vi "Verify and Check-In.vi"(0 "File Data Manager in":refnum<class "File Data Manager.lvclass">, 5 "Rooms Manager GUID":string, 7 "Room No":string, 9 "Guest Contact Number In":string caption="Guest Contact Number", 11 "error in (no error)":errorcluster, 12 "Primary Guest Name":string, 13 "Adults":u32, 14 "Children":u32) -> (4 "File Data Manager out":refnum<class "File Data Manager.lvclass">, 15 "error out":errorcluster)   [LabVIEW 2023, in "File Data Manager.lvlib" / "File Data Manager.lvclass"]
uses:
  File Data Manager.lvclass
  C:/Program Files/National Instruments/LabVIEW 2023/vi.lib/ActorFramework/Actor/Actor.lvclass
  File Data Manager.lvclass/File Data Manager.ctl
  Central Data Manager/Central Data Manager/Room Occupancy Status.ctl
  <vilib>/ActorFramework/Actor/Actor.lvclass/Actor.ctl
  <vilib>/ActorFramework/Message Enqueuer/Message Enqueuer.lvclass/Message Enqueuer.ctl
  Interfaces/Incoming Hotel Management Tool Model Interface Messages/Update Check-in Status Msg/Update Check-in Status Msg.lvclass/Update Check-in Status Msg.ctl
  <vilib>/ActorFramework/Message Enqueuer/Init from Existing Queue.vi
  <vilib>/ActorFramework/Message Enqueuer/Enqueue.vi
  Interfaces/Incoming Hotel Management Tool Model Interface Messages/Update Check-in Status Msg/Update Check-in Status Msg.lvclass
  C:/Program Files/National Instruments/LabVIEW 2023/vi.lib/ActorFramework/Message/Message.lvclass
  Central Data Manager/Central Data Manager Messages/Refresh Rooms Status Msg/Refresh Rooms Status Msg.lvclass
  <vilib>/ActorFramework/Message Priority Queue/Priority Enqueue.vi
  <vilib>/ActorFramework/Message Enqueuer/Message Enqueuer.lvclass
  Central Data Manager/Central Data Manager/Central Data Manager.lvclass
  <vilib>/ActorFramework/Actor/Actor.lvclass
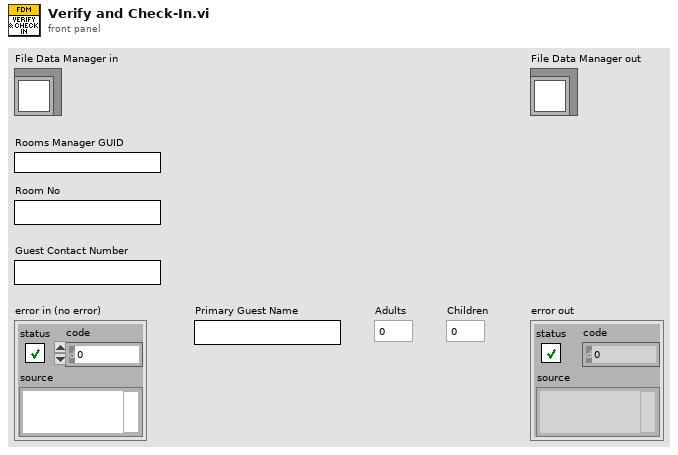
[diagram p1: front panel]
types:
  T1 = typedef "Central Data Manager.lvlib/Central Data Manager.lvclass/Room Occupancy Status.ctl" = enum16{"Not Occupied", "Occupied", "Under Maintainance", "Not Servicable"}
  T2 = typedef "Central Data Manager.lvlib/Central Data Manager.lvclass/Room Details.ctl" = cluster{"Room No":string, "Room Size":string, "Room Occupancy Status":T1, "Guest Details":T3, "Occupancy Count (Adult)":u32, "Occupancy Count (Children)":u32, "Check-in Time":timestamp, "Check-out Time":timestamp}
  T3 = typedef "Central Data Manager.lvlib/Central Data Manager.lvclass/Guest Details.ctl" = cluster{"Contact Number":string, "Primary Guest Name":string}
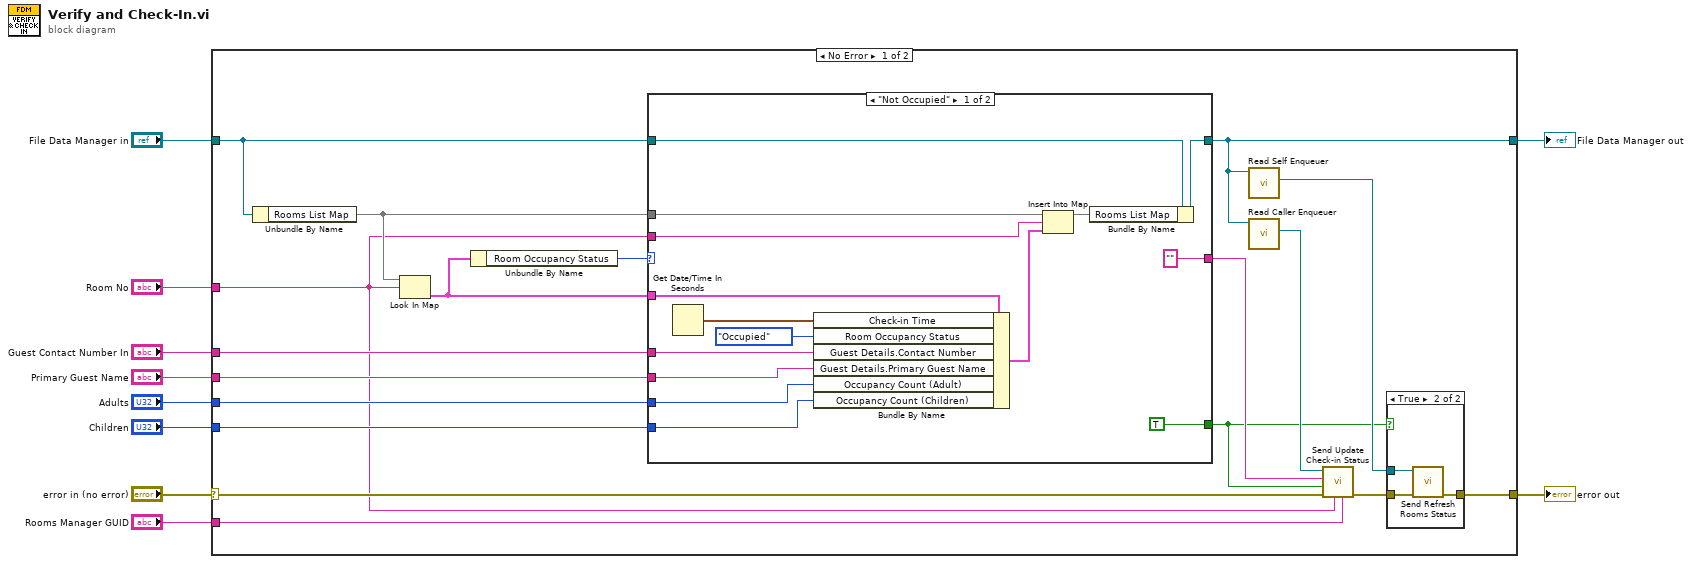
[diagram p0: block diagram]
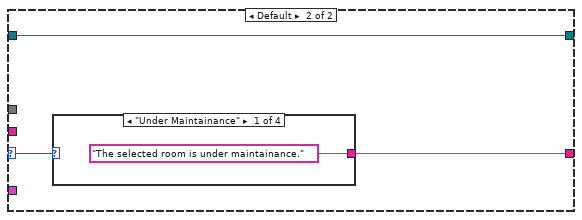
[diagram p3: hidden frame]
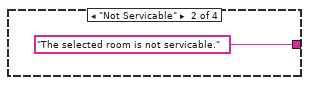
[diagram p4: hidden frame]
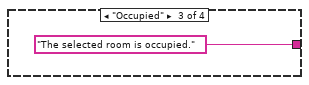
[diagram p5: hidden frame]
diagram:
  n1 = case shown="No Error" "error in (no error)" {
    selector: "error in (no error)" -> [w19 w54]
    tunnel: "File Data Manager in" -> [w26 w55]
    tunnel: "Guest Contact Number In" -> [w24 _]
    tunnel: "Primary Guest Name" -> [w23 _]
    tunnel: "Adults" -> [w22 _]
    tunnel: "Children" -> [w21 _]
    tunnel: "Room No" -> [w11 _]
    tunnel: [w15 w55] -> w4
    tunnel: "Rooms Manager GUID" -> [w12 _]
    tunnel: [w16 w54] -> w1
    frame No Error {
      n2 = Unbundle By Name(w26) -> ("Rooms List Map"=w25:map{string, T2})
      n3 = Look In Map(map=w25, key=w11) -> (value=w27:T2)  [unwired: 1 in, 1 out]
      n4 = Unbundle By Name(w27) -> ("Room Occupancy Status"=w28:T1)
      n5 = case shown="\"Not Occupied\"" w28 {
        selector: w28 -> [_ w49]
        tunnel: w27 -> [w43 _]
        tunnel: w26 -> [w47 w50]
        tunnel: [w46 w50] -> w15
        tunnel: w25 -> [w45 _]
        tunnel: w24 -> [w41 _]
        tunnel: w23 -> [w39 _]
        tunnel: w22 -> [w38 _]
        tunnel: w21 -> [w37 _]
        tunnel: w11 -> [w35 _]
        tunnel: ["" w48] -> w18
        tunnel: [TRUE _] -> w13
        frame "Not Occupied" {
          n6 = Get Date/Time In Seconds() -> (seconds since 1Jan1904=w40:timestamp)
          n7 = Bundle By Name(cluster=w43, "Check-in Time"=w40, "Room Occupancy Status"=Room_Occupancy_Status."Occupied", "Guest Details.Contact Number"=w41, "Guest Details.Primary Guest Name"=w39, "Occupancy Count (Adult)"=w38, "Occupancy Count (Children)"=w37) -> (w36:T2)
          n8 = Insert Into Map(map in=w45, key=w35, value=w36) -> (map out=w44:map{string, T2})  [unwired: 2 out]
          n9 = Bundle By Name(cluster=w47, "Rooms List Map"=w44) -> (w46:refnum<class "File Data Manager.lvclass">)
        }
        frame Default {
          n10 = case shown="\"Under Maintainance\"" w49 {
            tunnel: ["The selected room is under maintainance." "The selected room is not servicable." "The selected room is occupied." _] -> w48
            frame "Under Maintainance" {
            }
            frame "Not Servicable" {
            }
            frame "Occupied" {
            }
            frame Default {
            }
          }
        }
      }
      n11 = call <vilib>:"Read Self Enqueuer.vi"("Actor"=w15) -> ("Self Enqueuer"=w14:refnum<class "Message Enqueuer.lvclass">)  [unwired: 10 in]
      n12 = call <vilib>:"Read Caller Enqueuer.vi"("Actor"=w15) -> ("Caller Enqueuer"=w20:refnum<class "Message Enqueuer.lvclass">)  [unwired: 10 in]
      n13 = call "Send Update Check-in Status.vi"("Rooms Manager GUID"=w12, "Room No"=w11, "error in (no error)"=w19, "IsSuccess"=w13, "Reason If Failure"=w18, "Message Enqueuer"=w20) -> ("error out"=w17:errorcluster)  [unwired: 4 in, 1 out]
      n14 = case shown="True" w13 {
        tunnel: w17 -> [w29 w32]
        tunnel: [w29 w31] -> w16
        tunnel: w14 -> [_ w30]
        frame False {
        }
        frame True {
          n15 = call "Send Refresh Rooms Status.vi"("error in (no error)"=w32, "Message Enqueuer"=w30) -> ("error out"=w31:errorcluster)  [unwired: 8 in, 1 out]
        }
      }
    }
    frame Error {
    }
  }
  "error out" <- w1
  "File Data Manager out" <- w4
